vi "aFGV - MainPanel.vi"(6 "Action":T1, 8 "Error In":errorcluster, 9 "VI Ref":refnum<vi>, 11 "Main SubPanel Ref":refnum<vi>) -> (0 "Error Out":errorcluster, 2 "Event Active Page":refnum<user-event>, 3 "VI Name":string)   [LabVIEW 2020]
uses:
  Control/aFGV States - Subpanel.ctl
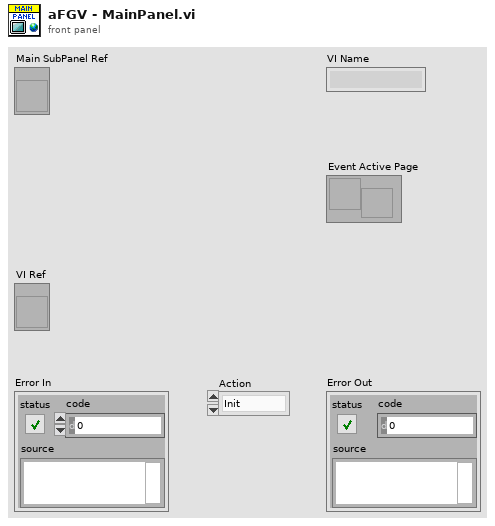
[diagram p1: front panel]
types:
  T1 = typedef "aFGV States - Subpanel.ctl" = enum16{"Init", "Get VI Name", "Update", "Exit"}
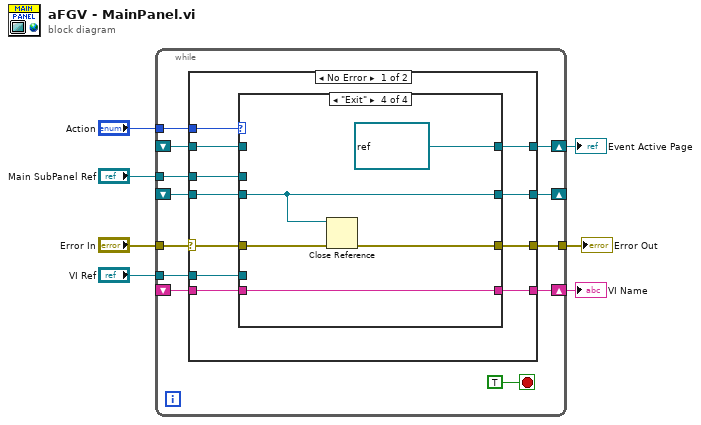
[diagram p0: block diagram]
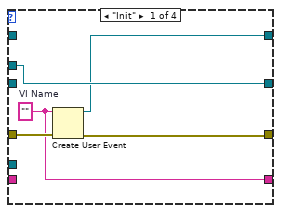
[diagram p2: hidden frame]
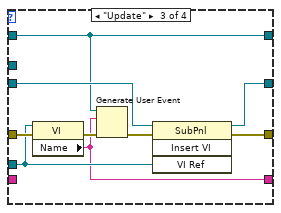
[diagram p4: hidden frame]
diagram:
  n1 = while {
    tunnel: [w19] -> w7
    tunnel: "Error In" -> [w18]
    tunnel: "Main SubPanel Ref" -> [w17]
    tunnel: "Action" -> [w15]
    shift-right: [w14] -> _
    shift-left: _ -> [w13]
    tunnel: "VI Ref" -> [w12]
    shift-right: [w10] -> w1
    shift-left: _ -> [w9]
    shift-right: [w11] -> w2
    shift-left: _ -> [w8]
    stop <- TRUE stop-if-true
    n2 = case shown="No Error" w18 {
      selector: w18 -> [w29 w57]
      tunnel: [w30 w57] -> w19
      tunnel: w17 -> [w28 _]
      tunnel: w15 -> [w27 _]
      tunnel: [w26 w56] -> w14
      tunnel: w13 -> [w25 w56]
      tunnel: w12 -> [w24 _]
      tunnel: [w23 w54] -> w11
      tunnel: [w22 w55] -> w10
      tunnel: w9 -> [w21 w55]
      tunnel: w8 -> [w20 w54]
      frame No Error {
        n3 = case shown="\"Exit\"" w27 {
          tunnel: [w35 w39 w48 w52] -> w30
          tunnel: w28 -> [w33 _ _ _]
          tunnel: w29 -> [w34 w39 w45 w53]
          tunnel: [w33 w38 w43 w51] -> w26
          tunnel: w25 -> [_ w38 w44 w51]
          tunnel: w24 -> [_ _ w42 _]
          tunnel: [w31 w36 w41 w50] -> w23
          tunnel: [w32 w37 w40 refnum<user-event> refnum ("VI Name")] -> w22
          tunnel: w21 -> [_ w37 w40 _]
          tunnel: w20 -> [_ w36 _ w50]
          frame "Init" {
            w31 = ""  # VI Name
            n4 = Create User Event(user event datatype=w31, error in=w34) -> (user event=w32:refnum<user-event>, error out=w35:errorcluster)
          }
          frame "Get VI Name" {
          }
          frame "Update" {
            n5 = property class="VI"(reference=w42, error in=w45) -> (error out=w47:errorcluster, "Name"=w41:string)  [unwired: 1 out]
            n6 = Generate User Event(user event=w40, event data cluster=w41, error in=w47) -> (error out=w46:errorcluster)  [unwired: 1 in, 1 out]
            n7 = invoke on="Invoke Node" class="SubPnl" method="Insert VI"(reference=w44, error in=w46, "VI Ref"=w42) -> (reference out=w43:refnum<vi>, error out=w48:errorcluster)  [unwired: 1 in, 2 out]
          }
          frame "Exit" {
            n8 = Close Reference(reference=w51, error in (no error)=w53) -> (error out=w52:errorcluster)
          }
        }
      }
      frame Error {
      }
    }
  }
  "Error Out" <- w7
  "VI Name" <- w2
  "Event Active Page" <- w1
